vi "S4GUI.vi"(7 "Tab ObsEng":enum32{"Obs", "CCD modes", "Guider", "Eng"}(tab)) -> ()   [LabVIEW 2018] (continued)
                n3564 = call-dynamic "Write Interface.vi"("error in (no error)"=w7905, "Interface.lvclass"=w7906, "Channel in"=w7921) -> ("error out"=w7902:errorcluster, "Channel out"=w7904:refnum<class "Channel.lvclass">)  [unwired: 7 in]
                n3565 = disable-structure shown="Enabled" {
                  disable-tunnel: w7904 -> [w7952 w7954]
                  disable-tunnel: [w7950 w7954] -> w7903
                  disable-tunnel: w7902 -> [w7949 w7953]
                  disable-tunnel: [w7944 w7953] -> w7901
                  frame Disabled {
                    n3566 = call-dynamic "Read State Machine.vi"("error in (no error)"=w7949, "Device in"=w7952) -> ("error out"=w7948:errorcluster, "State Machine.lvclass"=w7946:refnum<class "State Machine.lvclass">, "Device out"=w7951:refnum<class "Channel.lvclass">)  [unwired: 7 in]
                    n3567 = call "Next State.vi"("error in (no error)"=w7948, "New_State"=12, "State Machine in"=w7946) -> ("error out"=w7947:errorcluster, "State Machine out"=w7945:refnum<class "State Machine.lvclass">)  [unwired: 7 in]
                    n3568 = call-dynamic "Write State Machine.vi"("error in (no error)"=w7947, "State Machine.lvclass"=w7945, "Device in"=w7951) -> ("error out"=w7944:errorcluster, "Device out"=w7950:refnum<class "Channel.lvclass">)  [unwired: 7 in]
                  }
                  frame Enabled {
                  }
                }
                n3569 = call-dynamic "Write Channel.vi"("error in (no error)"=w7901, "Channel.lvclass"=w7903, "Acquisition in"=w7918) -> ("error out"=w7916:errorcluster, "Acquisition out"=w7917:refnum<class "Acquisition.lvclass">)  [unwired: 7 in]
                n3570 = call-dynamic "Write AcquisitionA.vi"("error in (no error)"=w7916, "Acquisition.lvclass"=w7917, "S4ACS_GUI in"=w7919) -> ("error out"=w7914:errorcluster, "S4ACS_GUI out"=w7915:refnum<class "S4GUI.lvclass">)  [unwired: 7 in]
              }
              frame #1 {
                # "suffix"
                n3571 = call "Read AcquisitionB.vi"("error in (no error)"=w7984, "S4ACS_GUI in"=w7985) -> ("error out"=w7972:errorcluster, "Acquisition.lvclass"=w7973:refnum<class "Acquisition.lvclass">, "S4ACS_GUI out"=w7976:refnum<class "S4GUI.lvclass">)  [unwired: 7 in]
                n3572 = call-dynamic "Read Channel.vi"("error in (no error)"=w7972, "Acquisition in"=w7973) -> ("error out"=w7956:errorcluster, "Channel.lvclass"=w7958:refnum<class "Channel.lvclass">, "Acquisition out"=w7977:refnum<class "Acquisition.lvclass">)  [unwired: 7 in]
                n3573 = local read "Filter2"() -> (w7959:u8)
                n3574 = call-dynamic "Write Filter.vi"("error in (no error)"=w7956, "Filter"=w7959, "Channel in"=w7958) -> ("error out"=w7955:errorcluster, "Channel out"=w7957:refnum<class "Channel.lvclass">)  [unwired: 7 in]
                n3575 = call-dynamic "Read Interface.vi"("error in (no error)"=w7955, "Channel in"=w7957) -> ("error out"=w7964:errorcluster, "Interface.lvclass"=w7965:refnum<class "Interface.lvclass">, "Channel out"=w7974:refnum<class "Channel.lvclass">)  [unwired: 7 in]
                n3576 = call-dynamic "Write Suffix.vi"("error in (no error)"=w7964, "Suffix"=w7981, "Interface in"=w7965) -> ("error out"=w7971:errorcluster, "Interface out"=w7975:refnum<class "Interface.lvclass">)  [unwired: 7 in]
                n3577 = disable-structure shown="Enabled" {
                  disable-tunnel: w7980 -> [w7999 _]
                  disable-tunnel: w7975 -> [w7996 w8001]
                  disable-tunnel: w7971 -> [w7993 w8000]
                  disable-tunnel: w7970 -> [w7992 _]
                  disable-tunnel: w7969 -> [w7991 _]
                  disable-tunnel: w7968 -> [w7990 _]
                  disable-tunnel: [w7989 w8001] -> w7967
                  disable-tunnel: [w7988 w8000] -> w7966
                  frame Disabled {
                    # "object"
                    # "obsType"
                    n3578 = call-dynamic "Write ObsType.vi"("error in (no error)"=w7993, "ObsType"=w7992, "Interface in"=w7996) -> ("error out"=w7994:errorcluster, "Interface out"=w7997:refnum<class "Interface.lvclass">)  [unwired: 7 in]
                    n3579 = call-dynamic "Write Object.vi"("error in (no error)"=w7994, "Object"=w7991, "Interface in"=w7997) -> ("error out"=w7995:errorcluster, "Interface out"=w7998:refnum<class "Interface.lvclass">)  [unwired: 7 in]
                    n3580 = call-dynamic "Write Comments.vi"("error in (no error)"=w7995, "Comments"=w7999, "Interface in"=w7998) -> ("error out"=w7987:errorcluster, "Interface out"=w7986:refnum<class "Interface.lvclass">)  [unwired: 7 in]
                    n3581 = call-dynamic "Write Observer.vi"("error in (no error)"=w7987, "Observer"=w7990, "Interface in"=w7986) -> ("error out"=w7988:errorcluster, "Interface out"=w7989:refnum<class "Interface.lvclass">)  [unwired: 7 in]
                  }
                  frame Enabled {
                  }
                }
                n3582 = call-dynamic "Write Interface.vi"("error in (no error)"=w7966, "Interface.lvclass"=w7967, "Channel in"=w7974) -> ("error out"=w7962:errorcluster, "Channel out"=w7963:refnum<class "Channel.lvclass">)  [unwired: 7 in]
                n3583 = disable-structure shown="Enabled" {
                  disable-tunnel: w7963 -> [w8006 w8013]
                  disable-tunnel: w7962 -> [w8005 w8012]
                  disable-tunnel: [w8003 w8013] -> w7961
                  disable-tunnel: [w8002 w8012] -> w7960
                  frame Disabled {
                    n3584 = call-dynamic "Read State Machine.vi"("error in (no error)"=w8005, "Device in"=w8006) -> ("error out"=w8011:errorcluster, "State Machine.lvclass"=w8009:refnum<class "State Machine.lvclass">, "Device out"=w8004:refnum<class "Channel.lvclass">)  [unwired: 7 in]
                    n3585 = call "Next State.vi"("error in (no error)"=w8011, "New_State"=12, "State Machine in"=w8009) -> ("error out"=w8010:errorcluster, "State Machine out"=w8008:refnum<class "State Machine.lvclass">)  [unwired: 7 in]
                    n3586 = call-dynamic "Write State Machine.vi"("error in (no error)"=w8010, "State Machine.lvclass"=w8008, "Device in"=w8004) -> ("error out"=w8002:errorcluster, "Device out"=w8003:refnum<class "Channel.lvclass">)  [unwired: 7 in]
                  }
                  frame Enabled {
                  }
                }
                n3587 = call-dynamic "Write Channel.vi"("error in (no error)"=w7960, "Channel.lvclass"=w7961, "Acquisition in"=w7977) -> ("error out"=w7979:errorcluster, "Acquisition out"=w7978:refnum<class "Acquisition.lvclass">)  [unwired: 7 in]
                n3588 = call "Write AcquisitionB.vi"("error in (no error)"=w7979, "Acquisition.lvclass"=w7978, "S4ACS_GUI in"=w7976) -> ("error out"=w7982:errorcluster, "S4ACS_GUI out"=w7983:refnum<class "S4GUI.lvclass">)  [unwired: 7 in]
              }
              frame #2 {
                # "suffix"
                n3589 = call-dynamic "Read AcquisitionC.vi"("error in (no error)"=w8043, "S4ACS_GUI in"=w8044) -> ("error out"=w8038:errorcluster, "Acquisition.lvclass"=w8037:refnum<class "Acquisition.lvclass">, "S4ACS_GUI out"=w8034:refnum<class "S4GUI.lvclass">)  [unwired: 7 in]
                n3590 = call-dynamic "Read Channel.vi"("error in (no error)"=w8038, "Acquisition in"=w8037) -> ("error out"=w8015:errorcluster, "Channel.lvclass"=w8017:refnum<class "Channel.lvclass">, "Acquisition out"=w8033:refnum<class "Acquisition.lvclass">)  [unwired: 7 in]
                n3591 = local read "Filter3"() -> (w8018:u8)
                n3592 = call-dynamic "Write Filter.vi"("error in (no error)"=w8015, "Filter"=w8018, "Channel in"=w8017) -> ("error out"=w8014:errorcluster, "Channel out"=w8016:refnum<class "Channel.lvclass">)  [unwired: 7 in]
                n3593 = call-dynamic "Read Interface.vi"("error in (no error)"=w8014, "Channel in"=w8016) -> ("error out"=w8025:errorcluster, "Interface.lvclass"=w8026:refnum<class "Interface.lvclass">, "Channel out"=w8036:refnum<class "Channel.lvclass">)  [unwired: 7 in]
                n3594 = call-dynamic "Write Suffix.vi"("error in (no error)"=w8025, "Suffix"=w8040, "Interface in"=w8026) -> ("error out"=w8039:errorcluster, "Interface out"=w8035:refnum<class "Interface.lvclass">)  [unwired: 7 in]
                n3595 = disable-structure shown="Enabled" {
                  disable-tunnel: w8039 -> [w8058 w8059]
                  disable-tunnel: w8035 -> [w8055 w8060]
                  disable-tunnel: w8030 -> [w8052 _]
                  disable-tunnel: w8029 -> [w8051 _]
                  disable-tunnel: w8028 -> [w8050 _]
                  disable-tunnel: w8027 -> [w8049 _]
                  disable-tunnel: [w8048 w8060] -> w8024
                  disable-tunnel: [w8047 w8059] -> w8023
                  frame Disabled {
                    # "object"
                    # "obsType"
                    n3596 = call-dynamic "Write ObsType.vi"("error in (no error)"=w8058, "ObsType"=w8051, "Interface in"=w8055) -> ("error out"=w8057:errorcluster, "Interface out"=w8054:refnum<class "Interface.lvclass">)  [unwired: 7 in]
                    n3597 = call-dynamic "Write Object.vi"("error in (no error)"=w8057, "Object"=w8050, "Interface in"=w8054) -> ("error out"=w8056:errorcluster, "Interface out"=w8053:refnum<class "Interface.lvclass">)  [unwired: 7 in]
                    n3598 = call-dynamic "Write Comments.vi"("error in (no error)"=w8056, "Comments"=w8052, "Interface in"=w8053) -> ("error out"=w8046:errorcluster, "Interface out"=w8045:refnum<class "Interface.lvclass">)  [unwired: 7 in]
                    n3599 = call-dynamic "Write Observer.vi"("error in (no error)"=w8046, "Observer"=w8049, "Interface in"=w8045) -> ("error out"=w8047:errorcluster, "Interface out"=w8048:refnum<class "Interface.lvclass">)  [unwired: 7 in]
                  }
                  frame Enabled {
                  }
                }
                n3600 = call-dynamic "Write Interface.vi"("error in (no error)"=w8023, "Interface.lvclass"=w8024, "Channel in"=w8036) -> ("error out"=w8021:errorcluster, "Channel out"=w8022:refnum<class "Channel.lvclass">)  [unwired: 7 in]
                n3601 = disable-structure shown="Enabled" {
                  disable-tunnel: w8022 -> [w8067 w8072]
                  disable-tunnel: w8021 -> [w8066 w8071]
                  disable-tunnel: [w8064 w8072] -> w8020
                  disable-tunnel: [w8061 w8071] -> w8019
                  frame Disabled {
                    n3602 = call-dynamic "Read State Machine.vi"("error in (no error)"=w8066, "Device in"=w8067) -> ("error out"=w8070:errorcluster, "State Machine.lvclass"=w8063:refnum<class "State Machine.lvclass">, "Device out"=w8065:refnum<class "Channel.lvclass">)  [unwired: 7 in]
                    n3603 = call "Next State.vi"("error in (no error)"=w8070, "New_State"=12, "State Machine in"=w8063) -> ("error out"=w8069:errorcluster, "State Machine out"=w8062:refnum<class "State Machine.lvclass">)  [unwired: 7 in]
                    n3604 = call-dynamic "Write State Machine.vi"("error in (no error)"=w8069, "State Machine.lvclass"=w8062, "Device in"=w8065) -> ("error out"=w8061:errorcluster, "Device out"=w8064:refnum<class "Channel.lvclass">)  [unwired: 7 in]
                  }
                  frame Enabled {
                  }
                }
                n3605 = call-dynamic "Write Channel.vi"("error in (no error)"=w8019, "Channel.lvclass"=w8020, "Acquisition in"=w8033) -> ("error out"=w8031:errorcluster, "Acquisition out"=w8032:refnum<class "Acquisition.lvclass">)  [unwired: 7 in]
                n3606 = call-dynamic "Write AcquisitionC.vi"("error in (no error)"=w8031, "Acquisition.lvclass"=w8032, "S4ACS_GUI in"=w8034) -> ("error out"=w8041:errorcluster, "S4ACS_GUI out"=w8042:refnum<class "S4GUI.lvclass">)  [unwired: 7 in]
              }
              frame #3 {
                # "suffix"
                n3607 = call-dynamic "Read AcquisitionD.vi"("error in (no error)"=w8102, "S4ACS_GUI in"=w8103) -> ("error out"=w8097:errorcluster, "Acquisition.lvclass"=w8096:refnum<class "Acquisition.lvclass">, "S4ACS_GUI out"=w8093:refnum<class "S4GUI.lvclass">)  [unwired: 7 in]
                n3608 = call-dynamic "Read Channel.vi"("error in (no error)"=w8097, "Acquisition in"=w8096) -> ("error out"=w8074:errorcluster, "Channel.lvclass"=w8076:refnum<class "Channel.lvclass">, "Acquisition out"=w8092:refnum<class "Acquisition.lvclass">)  [unwired: 7 in]
                n3609 = local read "Filter4"() -> (w8077:u8)
                n3610 = call-dynamic "Write Filter.vi"("error in (no error)"=w8074, "Filter"=w8077, "Channel in"=w8076) -> ("error out"=w8073:errorcluster, "Channel out"=w8075:refnum<class "Channel.lvclass">)  [unwired: 7 in]
                n3611 = call-dynamic "Read Interface.vi"("error in (no error)"=w8073, "Channel in"=w8075) -> ("error out"=w8084:errorcluster, "Interface.lvclass"=w8085:refnum<class "Interface.lvclass">, "Channel out"=w8095:refnum<class "Channel.lvclass">)  [unwired: 7 in]
                n3612 = call-dynamic "Write Suffix.vi"("error in (no error)"=w8084, "Suffix"=w8099, "Interface in"=w8085) -> ("error out"=w8098:errorcluster, "Interface out"=w8094:refnum<class "Interface.lvclass">)  [unwired: 7 in]
                n3613 = disable-structure shown="Enabled" {
                  disable-tunnel: w8098 -> [w8117 w8118]
                  disable-tunnel: w8094 -> [w8114 w8119]
                  disable-tunnel: w8089 -> [w8111 _]
                  disable-tunnel: w8088 -> [w8110 _]
                  disable-tunnel: w8087 -> [w8109 _]
                  disable-tunnel: w8086 -> [w8108 _]
                  disable-tunnel: [w8105 w8118] -> w8083
                  disable-tunnel: [w8104 w8119] -> w8082
                  frame Disabled {
                    # "object"
                    # "obsType"
                    n3614 = call-dynamic "Write ObsType.vi"("error in (no error)"=w8117, "ObsType"=w8110, "Interface in"=w8114) -> ("error out"=w8116:errorcluster, "Interface out"=w8113:refnum<class "Interface.lvclass">)  [unwired: 7 in]
                    n3615 = call-dynamic "Write Object.vi"("error in (no error)"=w8116, "Object"=w8109, "Interface in"=w8113) -> ("error out"=w8115:errorcluster, "Interface out"=w8112:refnum<class "Interface.lvclass">)  [unwired: 7 in]
                    n3616 = call-dynamic "Write Comments.vi"("error in (no error)"=w8115, "Comments"=w8111, "Interface in"=w8112) -> ("error out"=w8107:errorcluster, "Interface out"=w8106:refnum<class "Interface.lvclass">)  [unwired: 7 in]
                    n3617 = call-dynamic "Write Observer.vi"("error in (no error)"=w8107, "Observer"=w8108, "Interface in"=w8106) -> ("error out"=w8105:errorcluster, "Interface out"=w8104:refnum<class "Interface.lvclass">)  [unwired: 7 in]
                  }
                  frame Enabled {
                  }
                }
                n3618 = call-dynamic "Write Interface.vi"("error in (no error)"=w8083, "Interface.lvclass"=w8082, "Channel in"=w8095) -> ("error out"=w8079:errorcluster, "Channel out"=w8081:refnum<class "Channel.lvclass">)  [unwired: 7 in]
                n3619 = disable-structure shown="Enabled" {
                  disable-tunnel: w8081 -> [w8126 w8131]
                  disable-tunnel: [w8124 w8131] -> w8080
                  disable-tunnel: w8079 -> [w8123 w8130]
                  disable-tunnel: [w8122 w8130] -> w8078
                  frame Disabled {
                    n3620 = call-dynamic "Read State Machine.vi"("error in (no error)"=w8123, "Device in"=w8126) -> ("error out"=w8129:errorcluster, "State Machine.lvclass"=w8121:refnum<class "State Machine.lvclass">, "Device out"=w8125:refnum<class "Channel.lvclass">)  [unwired: 7 in]
                    n3621 = call "Next State.vi"("error in (no error)"=w8129, "New_State"=12, "State Machine in"=w8121) -> ("error out"=w8128:errorcluster, "State Machine out"=w8120:refnum<class "State Machine.lvclass">)  [unwired: 7 in]
                    n3622 = call-dynamic "Write State Machine.vi"("error in (no error)"=w8128, "State Machine.lvclass"=w8120, "Device in"=w8125) -> ("error out"=w8122:errorcluster, "Device out"=w8124:refnum<class "Channel.lvclass">)  [unwired: 7 in]
                  }
                  frame Enabled {
                  }
                }
                n3623 = call-dynamic "Write Channel.vi"("error in (no error)"=w8078, "Channel.lvclass"=w8080, "Acquisition in"=w8092) -> ("error out"=w8090:errorcluster, "Acquisition out"=w8091:refnum<class "Acquisition.lvclass">)  [unwired: 7 in]
                n3624 = call-dynamic "Write AcquisitionD.vi"("error in (no error)"=w8090, "Acquisition.lvclass"=w8091, "S4ACS_GUI in"=w8093) -> ("error out"=w8100:errorcluster, "S4ACS_GUI out"=w8101:refnum<class "S4GUI.lvclass">)  [unwired: 7 in]
              }
            }
          }
          frame True {
          }
        }
      }
      event "Observer": Mouse Enter {
        n3625 = event-data() -> ()  [unwired: 1 in, 4 out]
        n3626 = disable-structure shown="Disabled" {
          disable-tunnel: [w8139 w8142] -> w8135
          disable-tunnel: w8134 -> [w8137 w8142]
          frame Disabled {
            n3627 = property on="Observer" class="Str"() -> ("Value"=w8138:string)  [unwired: 2 in, 2 out]
            n3628 = String Length(string=w8138) -> (length=w8141:i32)
            n3629 = Equal To 0?(x=w8141) -> (x = 0?=w8140:bool)
            n3630 = property on="Observer" class="Str"(error in=w8137, "Caption.Visible"=w8140) -> (error out=w8139:errorcluster)  [unwired: 1 in, 1 out]
          }
          frame Enabled {
            # "Não se usa mais o texto de fundo\ndo controle \"Observer\""
          }
        }
      }
      event "Filter1", "Filter2", "Filter3", "Filter4": Value Change {
        n3631 = event-data() -> ()  [unwired: 1 in, 6 out]
        n3632 = stacked-sequence {
          seq-local: [w8173 _ _ _] -> [_ w8237 _ _]
          seq-local: [w8172 _ _ _] -> [_ w8236 _ _]
          seq-local: [_ w8235 _ _] -> [_ _ w8286 _]
          seq-local: [_ w8234 _ _] -> [_ _ w8285 _]
          seq-local: [_ _ w8284 _] -> [_ _ _ w8335]
          seq-local: [_ _ w8283 _] -> [_ _ _ w8334]
          tunnel: w8150 -> [w8185 _ _ _]
          tunnel: w8151 -> [w8184 _ _ _]
          tunnel: [_ _ _ w8333] -> w8144
          tunnel: [_ _ _ w8332] -> w8143
          tunnel: w8148 -> [w8171 w8233 w8282 w8331]
          tunnel: w8147 -> [w8170 w8232 w8268 w8317]
          tunnel: w8145 -> [w8169 w8218 w8267 w8316]
          tunnel: w8149 -> [w8168 w8217 w8266 w8315]
          tunnel: w8146 -> [w8167 w8216 w8265 w8314]
          frame #0 {
            # "observer"
            # "comment"
            # "object"
            # "suffix"
            # "obsType"
            n3633 = call-dynamic "Read AcquisitionA.vi"("error in (no error)"=w8185, "S4ACS_GUI in"=w8184) -> ("error out"=w8183:errorcluster, "Acquisition.lvclass"=w8182:refnum<class "Acquisition.lvclass">, "S4ACS_GUI out"=w8177:refnum<class "S4GUI.lvclass">)  [unwired: 7 in]
            n3634 = call-dynamic "Read Channel.vi"("error in (no error)"=w8183, "Acquisition in"=w8182) -> ("error out"=w8153:errorcluster, "Channel.lvclass"=w8156:refnum<class "Channel.lvclass">, "Acquisition out"=w8176:refnum<class "Acquisition.lvclass">)  [unwired: 7 in]
            n3635 = local read "Filter1"() -> (w8154:u8)
            n3636 = call-dynamic "Write Filter.vi"("error in (no error)"=w8153, "Filter"=w8154, "Channel in"=w8156) -> ("error out"=w8152:errorcluster, "Channel out"=w8155:refnum<class "Channel.lvclass">)  [unwired: 7 in]
            n3637 = call-dynamic "Read Interface.vi"("error in (no error)"=w8152, "Channel in"=w8155) -> ("error out"=w8163:errorcluster, "Interface.lvclass"=w8164:refnum<class "Interface.lvclass">, "Channel out"=w8181:refnum<class "Channel.lvclass">)  [unwired: 7 in]
            n3638 = call-dynamic "Write Suffix.vi"("error in (no error)"=w8163, "Suffix"=w8171, "Interface in"=w8164) -> ("error out"=w8188:errorcluster, "Interface out"=w8180:refnum<class "Interface.lvclass">)  [unwired: 7 in]
            n3639 = call-dynamic "Write ObsType.vi"("error in (no error)"=w8188, "ObsType"=w8169, "Interface in"=w8180) -> ("error out"=w8187:errorcluster, "Interface out"=w8179:refnum<class "Interface.lvclass">)  [unwired: 7 in]
            n3640 = call-dynamic "Write Object.vi"("error in (no error)"=w8187, "Object"=w8168, "Interface in"=w8179) -> ("error out"=w8186:errorcluster, "Interface out"=w8178:refnum<class "Interface.lvclass">)  [unwired: 7 in]
            n3641 = call-dynamic "Write Comments.vi"("error in (no error)"=w8186, "Comments"=w8170, "Interface in"=w8178) -> ("error out"=w8166:errorcluster, "Interface out"=w8165:refnum<class "Interface.lvclass">)  [unwired: 7 in]
            n3642 = call-dynamic "Write Observer.vi"("error in (no error)"=w8166, "Observer"=w8167, "Interface in"=w8165) -> ("error out"=w8161:errorcluster, "Interface out"=w8162:refnum<class "Interface.lvclass">)  [unwired: 7 in]
            n3643 = call-dynamic "Write Interface.vi"("error in (no error)"=w8161, "Interface.lvclass"=w8162, "Channel in"=w8181) -> ("error out"=w8158:errorcluster, "Channel out"=w8160:refnum<class "Channel.lvclass">)  [unwired: 7 in]
            n3644 = disable-structure shown="Enabled" {
              disable-tunnel: w8160 -> [w8198 w8200]
              disable-tunnel: [w8196 w8200] -> w8159
              disable-tunnel: w8158 -> [w8195 w8199]
              disable-tunnel: [w8190 w8199] -> w8157
              frame Disabled {
                n3645 = call-dynamic "Read State Machine.vi"("error in (no error)"=w8195, "Device in"=w8198) -> ("error out"=w8194:errorcluster, "State Machine.lvclass"=w8192:refnum<class "State Machine.lvclass">, "Device out"=w8197:refnum<class "Channel.lvclass">)  [unwired: 7 in]
                n3646 = call "Next State.vi"("error in (no error)"=w8194, "New_State"=12, "State Machine in"=w8192) -> ("error out"=w8193:errorcluster, "State Machine out"=w8191:refnum<class "State Machine.lvclass">)  [unwired: 7 in]
                n3647 = call-dynamic "Write State Machine.vi"("error in (no error)"=w8193, "State Machine.lvclass"=w8191, "Device in"=w8197) -> ("error out"=w8190:errorcluster, "Device out"=w8196:refnum<class "Channel.lvclass">)  [unwired: 7 in]
              }
              frame Enabled {
              }
            }
            n3648 = call-dynamic "Write Channel.vi"("error in (no error)"=w8157, "Channel.lvclass"=w8159, "Acquisition in"=w8176) -> ("error out"=w8174:errorcluster, "Acquisition out"=w8175:refnum<class "Acquisition.lvclass">)  [unwired: 7 in]
            n3649 = call-dynamic "Write AcquisitionA.vi"("error in (no error)"=w8174, "Acquisition.lvclass"=w8175, "S4ACS_GUI in"=w8177) -> ("error out"=w8172:errorcluster, "S4ACS_GUI out"=w8173:refnum<class "S4GUI.lvclass">)  [unwired: 7 in]
          }
          frame #1 {
            # "object"
            # "suffix"
            # "obsType"
            n3650 = call "Read AcquisitionB.vi"("error in (no error)"=w8236, "S4ACS_GUI in"=w8237) -> ("error out"=w8222:errorcluster, "Acquisition.lvclass"=w8223:refnum<class "Acquisition.lvclass">, "S4ACS_GUI out"=w8228:refnum<class "S4GUI.lvclass">)  [unwired: 7 in]
            n3651 = call-dynamic "Read Channel.vi"("error in (no error)"=w8222, "Acquisition in"=w8223) -> ("error out"=w8202:errorcluster, "Channel.lvclass"=w8204:refnum<class "Channel.lvclass">, "Acquisition out"=w8229:refnum<class "Acquisition.lvclass">)  [unwired: 7 in]
            n3652 = local read "Filter2"() -> (w8205:u8)
            n3653 = call-dynamic "Write Filter.vi"("error in (no error)"=w8202, "Filter"=w8205, "Channel in"=w8204) -> ("error out"=w8201:errorcluster, "Channel out"=w8203:refnum<class "Channel.lvclass">)  [unwired: 7 in]
            n3654 = call-dynamic "Read Interface.vi"("error in (no error)"=w8201, "Channel in"=w8203) -> ("error out"=w8210:errorcluster, "Interface.lvclass"=w8211:refnum<class "Interface.lvclass">, "Channel out"=w8224:refnum<class "Channel.lvclass">)  [unwired: 7 in]
            n3655 = call-dynamic "Write Suffix.vi"("error in (no error)"=w8210, "Suffix"=w8233, "Interface in"=w8211) -> ("error out"=w8219:errorcluster, "Interface out"=w8225:refnum<class "Interface.lvclass">)  [unwired: 7 in]
            n3656 = call-dynamic "Write ObsType.vi"("error in (no error)"=w8219, "ObsType"=w8218, "Interface in"=w8225) -> ("error out"=w8220:errorcluster, "Interface out"=w8226:refnum<class "Interface.lvclass">)  [unwired: 7 in]
            n3657 = call-dynamic "Write Object.vi"("error in (no error)"=w8220, "Object"=w8217, "Interface in"=w8226) -> ("error out"=w8221:errorcluster, "Interface out"=w8227:refnum<class "Interface.lvclass">)  [unwired: 7 in]
            n3658 = call-dynamic "Write Comments.vi"("error in (no error)"=w8221, "Comments"=w8232, "Interface in"=w8227) -> ("error out"=w8213:errorcluster, "Interface out"=w8212:refnum<class "Interface.lvclass">)  [unwired: 7 in]
            n3659 = call-dynamic "Write Observer.vi"("error in (no error)"=w8213, "Observer"=w8216, "Interface in"=w8212) -> ("error out"=w8214:errorcluster, "Interface out"=w8215:refnum<class "Interface.lvclass">)  [unwired: 7 in]
            n3660 = call-dynamic "Write Interface.vi"("error in (no error)"=w8214, "Interface.lvclass"=w8215, "Channel in"=w8224) -> ("error out"=w8208:errorcluster, "Channel out"=w8209:refnum<class "Channel.lvclass">)  [unwired: 7 in]
            n3661 = disable-structure shown="Enabled" {
              disable-tunnel: w8209 -> [w8242 w8249]
              disable-tunnel: w8208 -> [w8241 w8248]
              disable-tunnel: [w8239 w8249] -> w8207
              disable-tunnel: [w8238 w8248] -> w8206
              frame Disabled {
                n3662 = call-dynamic "Read State Machine.vi"("error in (no error)"=w8241, "Device in"=w8242) -> ("error out"=w8247:errorcluster, "State Machine.lvclass"=w8245:refnum<class "State Machine.lvclass">, "Device out"=w8240:refnum<class "Channel.lvclass">)  [unwired: 7 in]
                n3663 = call "Next State.vi"("error in (no error)"=w8247, "New_State"=12, "State Machine in"=w8245) -> ("error out"=w8246:errorcluster, "State Machine out"=w8244:refnum<class "State Machine.lvclass">)  [unwired: 7 in]
                n3664 = call-dynamic "Write State Machine.vi"("error in (no error)"=w8246, "State Machine.lvclass"=w8244, "Device in"=w8240) -> ("error out"=w8238:errorcluster, "Device out"=w8239:refnum<class "Channel.lvclass">)  [unwired: 7 in]
              }
              frame Enabled {
              }
            }
            n3665 = call-dynamic "Write Channel.vi"("error in (no error)"=w8206, "Channel.lvclass"=w8207, "Acquisition in"=w8229) -> ("error out"=w8231:errorcluster, "Acquisition out"=w8230:refnum<class "Acquisition.lvclass">)  [unwired: 7 in]
            n3666 = call "Write AcquisitionB.vi"("error in (no error)"=w8231, "Acquisition.lvclass"=w8230, "S4ACS_GUI in"=w8228) -> ("error out"=w8234:errorcluster, "S4ACS_GUI out"=w8235:refnum<class "S4GUI.lvclass">)  [unwired: 7 in]
          }
          frame #2 {
            # "object"
            # "suffix"
            # "obsType"
            n3667 = call-dynamic "Read AcquisitionC.vi"("error in (no error)"=w8285, "S4ACS_GUI in"=w8286) -> ("error out"=w8278:errorcluster, "Acquisition.lvclass"=w8277:refnum<class "Acquisition.lvclass">, "S4ACS_GUI out"=w8272:refnum<class "S4GUI.lvclass">)  [unwired: 7 in]
            n3668 = call-dynamic "Read Channel.vi"("error in (no error)"=w8278, "Acquisition in"=w8277) -> ("error out"=w8252:errorcluster, "Channel.lvclass"=w8254:refnum<class "Channel.lvclass">, "Acquisition out"=w8271:refnum<class "Acquisition.lvclass">)  [unwired: 7 in]
            n3669 = local read "Filter3"() -> (w8255:u8)
            n3670 = call-dynamic "Write Filter.vi"("error in (no error)"=w8252, "Filter"=w8255, "Channel in"=w8254) -> ("error out"=w8251:errorcluster, "Channel out"=w8253:refnum<class "Channel.lvclass">)  [unwired: 7 in]
            n3671 = call-dynamic "Read Interface.vi"("error in (no error)"=w8251, "Channel in"=w8253) -> ("error out"=w8263:errorcluster, "Interface.lvclass"=w8264:refnum<class "Interface.lvclass">, "Channel out"=w8276:refnum<class "Channel.lvclass">)  [unwired: 7 in]
            n3672 = call-dynamic "Write Suffix.vi"("error in (no error)"=w8263, "Suffix"=w8282, "Interface in"=w8264) -> ("error out"=w8281:errorcluster, "Interface out"=w8275:refnum<class "Interface.lvclass">)  [unwired: 7 in]
            n3673 = call-dynamic "Write ObsType.vi"("error in (no error)"=w8281, "ObsType"=w8267, "Interface in"=w8275) -> ("error out"=w8280:errorcluster, "Interface out"=w8274:refnum<class "Interface.lvclass">)  [unwired: 7 in]
            n3674 = call-dynamic "Write Object.vi"("error in (no error)"=w8280, "Object"=w8266, "Interface in"=w8274) -> ("error out"=w8279:errorcluster, "Interface out"=w8273:refnum<class "Interface.lvclass">)  [unwired: 7 in]
            n3675 = call-dynamic "Write Comments.vi"("error in (no error)"=w8279, "Comments"=w8268, "Interface in"=w8273) -> ("error out"=w8260:errorcluster, "Interface out"=w8259:refnum<class "Interface.lvclass">)  [unwired: 7 in]
            n3676 = call-dynamic "Write Observer.vi"("error in (no error)"=w8260, "Observer"=w8265, "Interface in"=w8259) -> ("error out"=w8261:errorcluster, "Interface out"=w8262:refnum<class "Interface.lvclass">)  [unwired: 7 in]
            n3677 = call-dynamic "Write Interface.vi"("error in (no error)"=w8261, "Interface.lvclass"=w8262, "Channel in"=w8276) -> ("error out"=w8257:errorcluster, "Channel out"=w8258:refnum<class "Channel.lvclass">)  [unwired: 7 in]
            n3678 = disable-structure shown="Enabled" {
              disable-tunnel: w8258 -> [w8293 w8298]
              disable-tunnel: w8257 -> [w8292 w8297]
              disable-tunnel: [w8287 w8297] -> w8256
              disable-tunnel: [w8290 w8298] -> w8250
              frame Disabled {
                n3679 = call-dynamic "Read State Machine.vi"("error in (no error)"=w8292, "Device in"=w8293) -> ("error out"=w8296:errorcluster, "State Machine.lvclass"=w8289:refnum<class "State Machine.lvclass">, "Device out"=w8291:refnum<class "Channel.lvclass">)  [unwired: 7 in]
                n3680 = call "Next State.vi"("error in (no error)"=w8296, "New_State"=12, "State Machine in"=w8289) -> ("error out"=w8295:errorcluster, "State Machine out"=w8288:refnum<class "State Machine.lvclass">)  [unwired: 7 in]
                n3681 = call-dynamic "Write State Machine.vi"("error in (no error)"=w8295, "State Machine.lvclass"=w8288, "Device in"=w8291) -> ("error out"=w8287:errorcluster, "Device out"=w8290:refnum<class "Channel.lvclass">)  [unwired: 7 in]
              }
              frame Enabled {
              }
            }
            n3682 = call-dynamic "Write Channel.vi"("error in (no error)"=w8256, "Channel.lvclass"=w8250, "Acquisition in"=w8271) -> ("error out"=w8269:errorcluster, "Acquisition out"=w8270:refnum<class "Acquisition.lvclass">)  [unwired: 7 in]
            n3683 = call-dynamic "Write AcquisitionC.vi"("error in (no error)"=w8269, "Acquisition.lvclass"=w8270, "S4ACS_GUI in"=w8272) -> ("error out"=w8283:errorcluster, "S4ACS_GUI out"=w8284:refnum<class "S4GUI.lvclass">)  [unwired: 7 in]
          }
          frame #3 {
            # "object"
            # "suffix"
            # "obsType"
            n3684 = call-dynamic "Read AcquisitionD.vi"("error in (no error)"=w8334, "S4ACS_GUI in"=w8335) -> ("error out"=w8327:errorcluster, "Acquisition.lvclass"=w8326:refnum<class "Acquisition.lvclass">, "S4ACS_GUI out"=w8321:refnum<class "S4GUI.lvclass">)  [unwired: 7 in]
            n3685 = call-dynamic "Read Channel.vi"("error in (no error)"=w8327, "Acquisition in"=w8326) -> ("error out"=w8300:errorcluster, "Channel.lvclass"=w8302:refnum<class "Channel.lvclass">, "Acquisition out"=w8320:refnum<class "Acquisition.lvclass">)  [unwired: 7 in]
            n3686 = local read "Filter4"() -> (w8303:u8)
            n3687 = call-dynamic "Write Filter.vi"("error in (no error)"=w8300, "Filter"=w8303, "Channel in"=w8302) -> ("error out"=w8299:errorcluster, "Channel out"=w8301:refnum<class "Channel.lvclass">)  [unwired: 7 in]
            n3688 = call-dynamic "Read Interface.vi"("error in (no error)"=w8299, "Channel in"=w8301) -> ("error out"=w8312:errorcluster, "Interface.lvclass"=w8313:refnum<class "Interface.lvclass">, "Channel out"=w8325:refnum<class "Channel.lvclass">)  [unwired: 7 in]
            n3689 = call-dynamic "Write Suffix.vi"("error in (no error)"=w8312, "Suffix"=w8331, "Interface in"=w8313) -> ("error out"=w8330:errorcluster, "Interface out"=w8324:refnum<class "Interface.lvclass">)  [unwired: 7 in]
            n3690 = call-dynamic "Write ObsType.vi"("error in (no error)"=w8330, "ObsType"=w8316, "Interface in"=w8324) -> ("error out"=w8329:errorcluster, "Interface out"=w8323:refnum<class "Interface.lvclass">)  [unwired: 7 in]
            n3691 = call-dynamic "Write Object.vi"("error in (no error)"=w8329, "Object"=w8315, "Interface in"=w8323) -> ("error out"=w8328:errorcluster, "Interface out"=w8322:refnum<class "Interface.lvclass">)  [unwired: 7 in]
            n3692 = call-dynamic "Write Comments.vi"("error in (no error)"=w8328, "Comments"=w8317, "Interface in"=w8322) -> ("error out"=w8311:errorcluster, "Interface out"=w8310:refnum<class "Interface.lvclass">)  [unwired: 7 in]
            n3693 = call-dynamic "Write Observer.vi"("error in (no error)"=w8311, "Observer"=w8314, "Interface in"=w8310) -> ("error out"=w8309:errorcluster, "Interface out"=w8308:refnum<class "Interface.lvclass">)  [unwired: 7 in]
            n3694 = call-dynamic "Write Interface.vi"("error in (no error)"=w8309, "Interface.lvclass"=w8308, "Channel in"=w8325) -> ("error out"=w8305:errorcluster, "Channel out"=w8307:refnum<class "Channel.lvclass">)  [unwired: 7 in]
            n3695 = disable-structure shown="Enabled" {
              disable-tunnel: w8307 -> [w8342 w8347]
              disable-tunnel: [w8340 w8347] -> w8306
              disable-tunnel: w8305 -> [w8339 w8346]
              disable-tunnel: [w8338 w8346] -> w8304
              frame Disabled {
                n3696 = call-dynamic "Read State Machine.vi"("error in (no error)"=w8339, "Device in"=w8342) -> ("error out"=w8345:errorcluster, "State Machine.lvclass"=w8337:refnum<class "State Machine.lvclass">, "Device out"=w8341:refnum<class "Channel.lvclass">)  [unwired: 7 in]
                n3697 = call "Next State.vi"("error in (no error)"=w8345, "New_State"=12, "State Machine in"=w8337) -> ("error out"=w8344:errorcluster, "State Machine out"=w8336:refnum<class "State Machine.lvclass">)  [unwired: 7 in]
                n3698 = call-dynamic "Write State Machine.vi"("error in (no error)"=w8344, "State Machine.lvclass"=w8336, "Device in"=w8341) -> ("error out"=w8338:errorcluster, "Device out"=w8340:refnum<class "Channel.lvclass">)  [unwired: 7 in]
              }
              frame Enabled {
              }
            }
            n3699 = call-dynamic "Write Channel.vi"("error in (no error)"=w8304, "Channel.lvclass"=w8306, "Acquisition in"=w8320) -> ("error out"=w8318:errorcluster, "Acquisition out"=w8319:refnum<class "Acquisition.lvclass">)  [unwired: 7 in]
            n3700 = call-dynamic "Write AcquisitionD.vi"("error in (no error)"=w8318, "Acquisition.lvclass"=w8319, "S4ACS_GUI in"=w8321) -> ("error out"=w8332:errorcluster, "S4ACS_GUI out"=w8333:refnum<class "S4GUI.lvclass">)  [unwired: 7 in]
          }
        }
      }
      event "Start ch1": Value Change {
        n3701 = event-data() -> ()  [unwired: 1 in, 6 out]
        n3702 = call "Read Instrument.lvclass.vi"("error in (no error)"=w8360, "S4ACS_GUI in"=w8362) -> ("error out"=w8363:errorcluster, "Instrument.lvclass"=w8364:refnum<class "Instrument.lvclass">, "S4ACS_GUI out"=w8361:refnum<class "S4GUI.lvclass">)  [unwired: 7 in]
        n3703 = call-dynamic "Read mode.vi"("error in (no error)"=w8363, "Instrument in"=w8364) -> ("error out"=w8359:errorcluster, "mode"=w8358:bool)  [unwired: 7 in, 1 out]
        n3704 = call-dynamic "Read AcquisitionA.vi"("error in (no error)"=w8359, "S4ACS_GUI in"=w8361) -> ("error out"=w8376:errorcluster, "Acquisition.lvclass"=w8377:refnum<class "Acquisition.lvclass">, "S4ACS_GUI out"=w8379:refnum<class "S4GUI.lvclass">)  [unwired: 7 in]
        n3705 = call-dynamic "Read Acq_state.vi"("error in (no error)"=w8376, "Acquisition in"=w8377) -> ("error out"=w8373:errorcluster, "Acq_state"=w8375:u32, "Acquisition out"=w8372:refnum<class "Acquisition.lvclass">)  [unwired: 7 in]
        n3706 = Not Equal?(x=w8375, y=u32 400) -> (x != y?=w8378:bool)
        n3707 = case shown="True" w8378 {
          tunnel: w8379 -> [w8392 w8431]
          tunnel: [w8392 w8422] -> w8371
          tunnel: [w8387 w8412] -> w8357
          tunnel: w8373 -> [w8394 w8425]
          tunnel: w8372 -> [w8397 w8421]
          tunnel: [w8388 w8413] -> w8370
          tunnel: w8369 -> [_ w8444]
          tunnel: w8368 -> [_ w8443]
          tunnel: w8367 -> [_ w8442]
          tunnel: w8366 -> [_ w8441]
          tunnel: w8365 -> [_ w8436]
          tunnel: w8358 -> [_ _]
          tunnel: w8356 -> [_ w8416]
          tunnel: w8355 -> [_ w8419]
          tunnel: w8354 -> [_ w8418]
          tunnel: w8353 -> [_ w8417]
          frame False {
            n3708 = call-dynamic "Read Acq_prevstate.vi"("error in (no error)"=w8394, "Acquisition in"=w8397) -> ("error out"=w8393:errorcluster, "Acq_prevstate"=w8395:u32, "Acquisition out"=w8396:refnum<class "Acquisition.lvclass">)  [unwired: 7 in]
            n3709 = call-dynamic "Write Acq_state.vi"("error in (no error)"=w8393, "Acq_state"=w8395, "Acquisition in"=w8396) -> ("error out"=w8384:errorcluster, "Acquisition out"=w8386:refnum<class "Acquisition.lvclass">)  [unwired: 7 in]
            n3710 = call-dynamic "Read enabled.vi"("error in (no error)"=w8384, "Server in"=w8386) -> ("error out"=w8383:errorcluster, "enabled"=w8380:bool, "Server out"=w8385:refnum<class "Acquisition.lvclass">)  [unwired: 7 in]
            n3711 = call-dynamic "Read Channel.vi"("error in (no error)"=w8383, "Acquisition in"=w8385) -> ("error out"=w8381:errorcluster, "Channel.lvclass"=w8382:refnum<class "Channel.lvclass">, "Acquisition out"=w8391:refnum<class "Acquisition.lvclass">)  [unwired: 7 in]
            n3712 = case shown="True" w8380 {
              tunnel: w8382 -> [w8399 w8409]
              tunnel: [w8399 w8407] -> w8390
              tunnel: w8381 -> [w8398 w8404]
              tunnel: [w8398 w8402] -> w8389
              frame False {
              }
              frame True {
                n3713 = call-dynamic "Read State Machine.vi"("error in (no error)"=w8404, "Device in"=w8409) -> ("error out"=w8400:errorcluster, "State Machine.lvclass"=w8401:refnum<class "State Machine.lvclass">, "Device out"=w8408:refnum<class "Channel.lvclass">)  [unwired: 7 in]
                n3714 = call "Next State.vi"("error in (no error)"=w8400, "New_State"=96, "State Machine in"=w8401) -> ("error out"=w8403:errorcluster, "State Machine out"=w8406:refnum<class "State Machine.lvclass">)  [unwired: 7 in]
                n3715 = call-dynamic "Write State Machine.vi"("error in (no error)"=w8403, "State Machine.lvclass"=w8406, "Device in"=w8408) -> ("error out"=w8402:errorcluster, "Device out"=w8407:refnum<class "Channel.lvclass">)  [unwired: 7 in]
              }
            }
            n3716 = call-dynamic "Write Channel.vi"("error in (no error)"=w8389, "Channel.lvclass"=w8390, "Acquisition in"=w8391) -> ("error out"=w8387:errorcluster, "Acquisition out"=w8388:refnum<class "Acquisition.lvclass">)  [unwired: 7 in]
          }
          frame True {
            # "vide S4GUI:\nHandleObservationAsync.vi"
            # "object"
            # "suffix"
            # "obsType"
            n3717 = call "Read Instrument.lvclass.vi"("S4ACS_GUI in"=w8431) -> ("error out"=w8433:errorcluster, "Instrument.lvclass"=w8435:refnum<class "Instrument.lvclass">, "S4ACS_GUI out"=w8423:refnum<class "S4GUI.lvclass">)  [unwired: 8 in]
            n3718 = call "Read WPROT.vi"("error in (no error)"=w8433, "Instrument in"=w8435) -> ("error out"=w8432:errorcluster, "Opt_Selector.lvclass"=w8434:refnum<class "Opt_Selector.lvclass">)  [unwired: 7 in, 1 out]
            n3719 = call-dynamic "Read sequencia.vi"("error in (no error)"=w8432, "Opt_Selector in"=w8434) -> ()  [unwired: 7 in, 3 out]
            n3720 = case shown="\"FOCUS\"" w8416 {
              tunnel: [u32 271 ("Obs_state") u32 251 ("Obs_state")] -> w8424
              tunnel: w8425 -> [w8467 w8478]
              tunnel: [w8466 w8478] -> w8420
              tunnel: w8419 -> [w8474 _]
              tunnel: w8418 -> [w8473 _]
              tunnel: w8417 -> [w8472 _]
              tunnel: w8423 -> [w8465 w8477]
              tunnel: [w8464 w8477] -> w8422
              frame "FOCUS" {
                n3721 = call-dynamic "Read TelFocus.lvclass.vi"("error in (no error)"=w8467, "S4GUI in"=w8465) -> ("error out"=w8469:errorcluster, "TelFocus.lvclass"=w8471:refnum<class "TelFocus.lvclass">, "S4GUI out"=w8475:refnum<class "S4GUI.lvclass">)  [unwired: 7 in]
                n3722 = call-dynamic "LoadParam.vi"("#steps"=w8472, "error in (no error)"=w8469, "step"=w8473, "init"=w8474, "TelFocus in"=w8471) -> ("error out"=w8468:errorcluster, "TelFocus out"=w8470:refnum<class "TelFocus.lvclass">)  [unwired: 5 in]
                n3723 = call-dynamic "Write TelFocus.lvclass.vi"("error in (no error)"=w8468, "TelFocus.lvclass"=w8470, "S4GUI in"=w8475) -> ("error out"=w8466:errorcluster, "S4GUI out"=w8464:refnum<class "S4GUI.lvclass">)  [unwired: 7 in]
              }
              frame Default {
              }
            }
            n3724 = property on="Start ch1" class="Bool"(error in=w8425, "DisabledEnum"=T12."Disabled and Grayed Out" ("Disabled")) -> ()  [unwired: 1 in, 2 out]
            n3725 = call-dynamic "Write Acq_state.vi"("error in (no error)"=w8420, "Acq_state"=w8424, "Acquisition in"=w8421) -> ("error out"=w8445:errorcluster, "Acquisition out"=w8446:refnum<class "Acquisition.lvclass">)  [unwired: 7 in]
            n3726 = call-dynamic "Read Channel.vi"("error in (no error)"=w8445, "Acquisition in"=w8446) -> ("error out"=w8447:errorcluster, "Channel.lvclass"=w8448:refnum<class "Channel.lvclass">, "Acquisition out"=w8452:refnum<class "Acquisition.lvclass">)  [unwired: 7 in]
            n3727 = call-dynamic "Read Interface.vi"("error in (no error)"=w8447, "Channel in"=w8448) -> ("error out"=w8462:errorcluster, "Interface.lvclass"=w8463:refnum<class "Interface.lvclass">, "Channel out"=w8461:refnum<class "Channel.lvclass">)  [unwired: 7 in]
            n3728 = call "Write Exposure Time.vi"("error in (no error)"=w8462, "Exposure Time"="Exptime ch1", "Interface in"=w8463) -> ("error out"=w8429:errorcluster, "Interface out"=w8430:refnum<class "Interface.lvclass">)  [unwired: 7 in]
            n3729 = case shown="Default" w8416 {
              tunnel: w8430 -> [w8481 w8486]
              tunnel: w8429 -> [w8480 w8485]
              tunnel: "Exptime ch1" -> [_ w8484]
              tunnel: [w8480 w8483] -> w8427
              tunnel: [w8481 w8482] -> w8426
              frame "ZERO" {
              }
              frame Default {
                n3730 = call-dynamic "Write prev ExpTime.vi"("error in (no error)"=w8485, "prev ExpTime"=w8484, "Interface in"=w8486) -> ("error out"=w8483:errorcluster, "Interface out"=w8482:refnum<class "Interface.lvclass">)  [unwired: 7 in]
              }
            }
            n3731 = call-dynamic "Write Suffix.vi"("error in (no error)"=w8427, "Suffix"=w8444, "Interface in"=w8426) -> ("error out"=w8460:errorcluster, "Interface out"=w8459:refnum<class "Interface.lvclass">)  [unwired: 7 in]
            n3732 = call-dynamic "Write ObsType.vi"("error in (no error)"=w8460, "ObsType"=w8442, "Interface in"=w8459) -> ("error out"=w8457:errorcluster, "Interface out"=w8458:refnum<class "Interface.lvclass">)  [unwired: 7 in]
            n3733 = call-dynamic "Write Object.vi"("error in (no error)"=w8457, "Object"=w8441, "Interface in"=w8458) -> ("error out"=w8456:errorcluster, "Interface out"=w8455:refnum<class "Interface.lvclass">)  [unwired: 7 in]
            n3734 = call-dynamic "Write Comments.vi"("error in (no error)"=w8456, "Comments"=w8443, "Interface in"=w8455) -> ("error out"=w8453:errorcluster, "Interface out"=w8454:refnum<class "Interface.lvclass">)  [unwired: 7 in]
            n3735 = call-dynamic "Write DS9.vi"("error in (no error)"=w8453, "DS9"="F", "Interface in"=w8454) -> ("error out"=w8438:errorcluster, "Interface out"=w8440:refnum<class "Interface.lvclass">)  [unwired: 7 in]
            n3736 = call-dynamic "Write Observer.vi"("error in (no error)"=w8438, "Observer"=w8436, "Interface in"=w8440) -> ("error out"=w8437:errorcluster, "Interface out"=w8439:refnum<class "Interface.lvclass">)  [unwired: 7 in]
            n3737 = call-dynamic "Write Interface.vi"("error in (no error)"=w8437, "Interface.lvclass"=w8439, "Channel in"=w8461) -> ("error out"=w8410:errorcluster, "Channel out"=w8411:refnum<class "Channel.lvclass">)  [unwired: 7 in]
            n3738 = property on="Exposure Time ch1" class="Slide (strict)"("Scale.Maximum"="Exptime ch1", "Scale.Minimum"=0.0 ("Scale.Range:Minimum")) -> ()  [unwired: 2 in, 2 out]
            n3739 = call-dynamic "Write Channel.vi"("error in (no error)"=w8410, "Channel.lvclass"=w8411, "Acquisition in"=w8452) -> ("error out"=w8414:errorcluster, "Acquisition out"=w8415:refnum<class "Acquisition.lvclass">)  [unwired: 7 in]
            n3740 = call-dynamic "CalcCubeDuration.vi"("error in (no error)"=w8414, "Acquisition in"=w8415) -> ("error out"=w8412:errorcluster, "Acquisition out"=w8413:refnum<class "Acquisition.lvclass">)  [unwired: 8 in]
          }
        }
        n3741 = call-dynamic "Write AcquisitionA.vi"("error in (no error)"=w8357, "Acquisition.lvclass"=w8370, "S4ACS_GUI in"=w8371) -> ("error out"=w8350:errorcluster, "S4ACS_GUI out"=w8351:refnum<class "S4GUI.lvclass">)  [unwired: 7 in]
        n3742 = call-dynamic "Write User Event.vi"("error in (no error)"=w8350, "User Event"="START ASYNC CH1", "S4GUI in"=w8351) -> ("error out"=w8348:errorcluster, "S4GUI out"=w8349:refnum<class "S4GUI.lvclass">)  [unwired: 7 in]
      }
      event "Exp ch1", "Exp ch2", "Exp ch3", "Exp ch4": Value Change {
        n3743 = event-data() -> ()  [unwired: 1 in, 6 out]
        n3744 = call-dynamic "Read AcquisitionA.vi"("error in (no error)"=w8591, "S4ACS_GUI in"=w8592) -> ("error out"=w8581:errorcluster, "Acquisition.lvclass"=w8589:refnum<class "Acquisition.lvclass">, "S4ACS_GUI out"=w8590:refnum<class "S4GUI.lvclass">)  [unwired: 7 in]
        n3745 = call-dynamic "Read Channel.vi"("error in (no error)"=w8581, "Acquisition in"=w8589) -> ("error out"=w8582:errorcluster, "Channel.lvclass"=w8588:refnum<class "Channel.lvclass">, "Acquisition out"=w8587:refnum<class "Acquisition.lvclass">)  [unwired: 7 in]
        n3746 = call-dynamic "Read Interface.vi"("error in (no error)"=w8582, "Channel in"=w8588) -> ("error out"=w8580:errorcluster, "Interface.lvclass"=w8583:refnum<class "Interface.lvclass">, "Channel out"=w8585:refnum<class "Channel.lvclass">)  [unwired: 7 in]
        n3747 = call-dynamic "Write # Images.vi"("error in (no error)"=w8580, "# Images"="Exp ch1", "Interface in"=w8583) -> ("error out"=w8509:errorcluster, "Interface out"=w8511:refnum<class "Interface.lvclass">)  [unwired: 7 in]
        n3748 = call-dynamic "ValidateExp.vi"("error in (no error)"=w8509, "Interface in"=w8511) -> ("error out"=w8508:errorcluster, "Interface out"=w8510:refnum<class "Interface.lvclass">)  [unwired: 8 in]
        n3749 = call-dynamic "Read # Images.vi"("error in (no error)"=w8508, "Interface in"=w8510) -> ("error out"=w8512:errorcluster, "# Images"=w8514:u32, "Interface out"=w8513:refnum<class "Interface.lvclass">)  [unwired: 7 in]
        n3750 = call-dynamic "Write #PREV Images.vi"("error in (no error)"=w8512, "#PREV FRAMES"=w8514, "Interface in"=w8513) -> ("error out"=w8579:errorcluster, "Interface out"=w8578:refnum<class "Interface.lvclass">)  [unwired: 7 in]
        n3751 = call-dynamic "Write Interface.vi"("error in (no error)"=w8579, "Interface.lvclass"=w8578, "Channel in"=w8585) -> ("error out"=w8577:errorcluster, "Channel out"=w8584:refnum<class "Channel.lvclass">)  [unwired: 7 in]
        n3752 = local write "Exp ch1"(w8514) -> ()
        n3753 = property on="Exposures Done ch1" class="Slide (strict)"("Scale.Maximum"=w8514, "Scale.Minimum"=0.0 ("Scale.Range:Minimum")) -> ()  [unwired: 2 in, 2 out]
        n3754 = call-dynamic "Write Channel.vi"("error in (no error)"=w8577, "Channel.lvclass"=w8584, "Acquisition in"=w8587) -> ("error out"=w8576:errorcluster, "Acquisition out"=w8586:refnum<class "Acquisition.lvclass">)  [unwired: 7 in]
        n3755 = call-dynamic "Write AcquisitionA.vi"("error in (no error)"=w8576, "Acquisition.lvclass"=w8586, "S4ACS_GUI in"=w8590) -> ("error out"=w8524:errorcluster, "S4ACS_GUI out"=w8525:refnum<class "S4GUI.lvclass">)  [unwired: 7 in]
        n3756 = call "Read AcquisitionB.vi"("error in (no error)"=w8524, "S4ACS_GUI in"=w8525) -> ("error out"=w8565:errorcluster, "Acquisition.lvclass"=w8573:refnum<class "Acquisition.lvclass">, "S4ACS_GUI out"=w8574:refnum<class "S4GUI.lvclass">)  [unwired: 7 in]
        n3757 = call-dynamic "Read Channel.vi"("error in (no error)"=w8565, "Acquisition in"=w8573) -> ("error out"=w8566:errorcluster, "Channel.lvclass"=w8572:refnum<class "Channel.lvclass">, "Acquisition out"=w8571:refnum<class "Acquisition.lvclass">)  [unwired: 7 in]
        n3758 = call-dynamic "Read Interface.vi"("error in (no error)"=w8566, "Channel in"=w8572) -> ("error out"=w8564:errorcluster, "Interface.lvclass"=w8567:refnum<class "Interface.lvclass">, "Channel out"=w8569:refnum<class "Channel.lvclass">)  [unwired: 7 in]
        n3759 = call-dynamic "Write # Images.vi"("error in (no error)"=w8564, "# Images"="Exp ch2", "Interface in"=w8567) -> ("error out"=w8505:errorcluster, "Interface out"=w8507:refnum<class "Interface.lvclass">)  [unwired: 7 in]
        n3760 = call-dynamic "ValidateExp.vi"("error in (no error)"=w8505, "Interface in"=w8507) -> ("error out"=w8504:errorcluster, "Interface out"=w8506:refnum<class "Interface.lvclass">)  [unwired: 8 in]
        n3761 = call-dynamic "Read # Images.vi"("error in (no error)"=w8504, "Interface in"=w8506) -> ("error out"=w8501:errorcluster, "# Images"=w8502:u32, "Interface out"=w8503:refnum<class "Interface.lvclass">)  [unwired: 7 in]
        n3762 = call-dynamic "Write #PREV Images.vi"("error in (no error)"=w8501, "#PREV FRAMES"=w8502, "Interface in"=w8503) -> ("error out"=w8563:errorcluster, "Interface out"=w8562:refnum<class "Interface.lvclass">)  [unwired: 7 in]
        n3763 = local write "Exp ch2"(w8502) -> ()
        n3764 = property on="Exposures Done ch2" class="Slide (strict)"("Scale.Maximum"=w8502, "Scale.Minimum"=0.0 ("Scale.Range:Minimum")) -> ()  [unwired: 2 in, 2 out]
        n3765 = call-dynamic "Write Interface.vi"("error in (no error)"=w8563, "Interface.lvclass"=w8562, "Channel in"=w8569) -> ("error out"=w8561:errorcluster, "Channel out"=w8568:refnum<class "Channel.lvclass">)  [unwired: 7 in]
        n3766 = call-dynamic "Write Channel.vi"("error in (no error)"=w8561, "Channel.lvclass"=w8568, "Acquisition in"=w8571) -> ("error out"=w8560:errorcluster, "Acquisition out"=w8570:refnum<class "Acquisition.lvclass">)  [unwired: 7 in]
        n3767 = call "Write AcquisitionB.vi"("error in (no error)"=w8560, "Acquisition.lvclass"=w8570, "S4ACS_GUI in"=w8574) -> ("error out"=w8526:errorcluster, "S4ACS_GUI out"=w8527:refnum<class "S4GUI.lvclass">)  [unwired: 7 in]
        n3768 = call-dynamic "Read AcquisitionC.vi"("error in (no error)"=w8526, "S4ACS_GUI in"=w8527) -> ("error out"=w8550:errorcluster, "Acquisition.lvclass"=w8558:refnum<class "Acquisition.lvclass">, "S4ACS_GUI out"=w8559:refnum<class "S4GUI.lvclass">)  [unwired: 7 in]
        n3769 = call-dynamic "Read Channel.vi"("error in (no error)"=w8550, "Acquisition in"=w8558) -> ("error out"=w8551:errorcluster, "Channel.lvclass"=w8557:refnum<class "Channel.lvclass">, "Acquisition out"=w8556:refnum<class "Acquisition.lvclass">)  [unwired: 7 in]
        n3770 = call-dynamic "Read Interface.vi"("error in (no error)"=w8551, "Channel in"=w8557) -> ("error out"=w8549:errorcluster, "Interface.lvclass"=w8552:refnum<class "Interface.lvclass">, "Channel out"=w8554:refnum<class "Channel.lvclass">)  [unwired: 7 in]
